vi "Kommandos einwerfen.vi"(10 "Zeitstempeln":timestamp[](array[timestamp])) -> (2 "Zeitstempeln":timestamp[](array[timestamp]), 5 "Kommandos":string[](array[string]))   [LabVIEW 2020, in "FT-IR.lvlib" / "AK-Interface.lvlib"]
uses:
  AK-Interface.lvlib
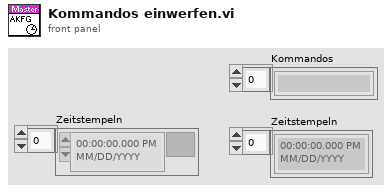
[diagram p1: front panel]
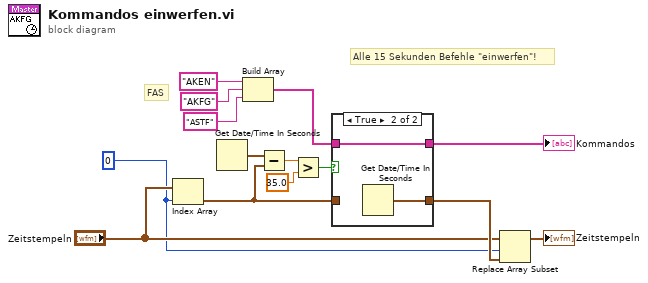
[diagram p0: block diagram]
diagram:
  w2 = 0 ("Index")
  # "Alle 15 Sekunden Befehle \"einwerfen\"!"
  # "FAS"
  n1 = Index Array(array="Zeitstempeln", index=w2) -> (element=w11:timestamp)
  n2 = Get Date/Time In Seconds() -> (seconds since 1Jan1904=w7:timestamp)
  n3 = Build Array("AKEN", "AKFG", "ASTF") -> (w5:string[])
  n4 = Subtract(x=w7, y=w11) -> (x-y=w8:dbl)
  n5 = Greater?(x=w8, y=35.0) -> (0:w10:bool)
  n6 = case shown="True" w10 {
    tunnel: w11 -> [w15 _]
    tunnel: [w15 w17] -> w13
    tunnel: [_ w16] -> w6
    tunnel: w5 -> [_ w16]
    frame False {
    }
    frame True {
      n7 = Get Date/Time In Seconds() -> (seconds since 1Jan1904=w17:timestamp)
    }
  }
  "Kommandos" <- w6
  n8 = Replace Array Subset(array="Zeitstempeln", new element=w13, index=w2) -> (→"Zeitstempeln":timestamp[])
